vi "Waveform Array to 2D Double.vi"(7 "Waveform []":waveform(dbl)[](array[waveform])) -> (6 "Y []":dbl[][](array[numeric]), 10 "dt":dbl)   [LabVIEW 2019]
doc: "Convert Waveform Array to 2D Double Array."
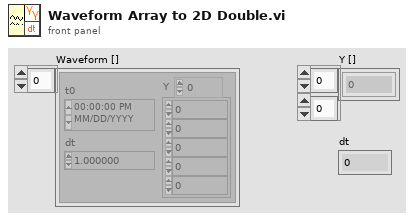
[diagram p1: front panel]
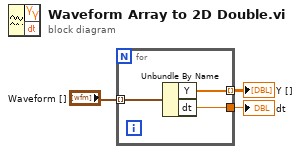
[diagram p0: block diagram]
diagram:
  n1 = for {
    tunnel: "Waveform []" -> [w6] mode=indexing
    tunnel: [w5] -> w2 mode=indexing
    tunnel: [w4] -> w1
    n2 = Unbundle By Name(w6) -> ("Y"=w5:dbl[], "dt"=w4:dbl)
  }
  "Y []" <- w2
  "dt" <- w1
